vi "Fdx Create UDP Port (RX-CommPort).vi"(8 "error in":errorcluster, 9 "VlId":u16, 10 "CommPort Config":T2={"PortType"=enum."FDX_UDP_SAMPLING", "SubVIId"=1, "domainID"=1, "sideID"=1, "locationID"=1, "partitionID"=1, "UdpSrcPort"=1, "UdpDstPort"=1, "UdpNumBufMessages"=0, "UdpMaxMessageSize"=1000, "UdpSamplingRate"=0} {"partitionID" format="%.0b"}, 11 "port handle in":u32) -> (0 "error out":errorcluster, 1 "computedAddresses":T1 {"MACsrc" format="%.0x"}, 2 "commPort handle out":u32, 3 "port handle out":u32)   [LabVIEW 2020, in "AIM664LV.lvlib"]
doc: "This function creates a port to receive data from a specified UDP connection oriented port.\n\nThis function can be used only if the receiver is not running. This function assumes that FdxCmdRxVLControl was previously called in order to enable a VL for reception. On this VL this function creates an FDX communication Rx-port.\n\n<B>subVLid</B>: Not relevant in Rx Mode\n<B>UdpNumBuffMessages</B>: Number of messages which should be stored. For sampling port number should be set to 1, while for queuing port it should be set to adequate value. If set to 0, onboard target software will be set to a default value.\n<B>UdpMaxMessageSiize</B>: maximum size of the messsage to be received. For a sampling port, this is the fixed size of the sampling message, which means the size without the header overhead (MAC, IP and UDP).\nFor a queuing port this is the maximum size of the variable length message.\n(Queuing: 0..ize ? 8kBytes, Sampling: ul_UdpMaxMessageSize )\n<B>UdpSamplliingRate</B>: not relevant in RX mode"
uses:
  AIM664LV.lvlib
  _controls/comm_udp_rx.ctl
  _controls/comm_computedMAC-IP.ctl
  helpers/EthFrameManagement/controls/ip_src_info_afdx.ctl
  helpers/EthFrameManagement/EthFrameManagement.lvlib
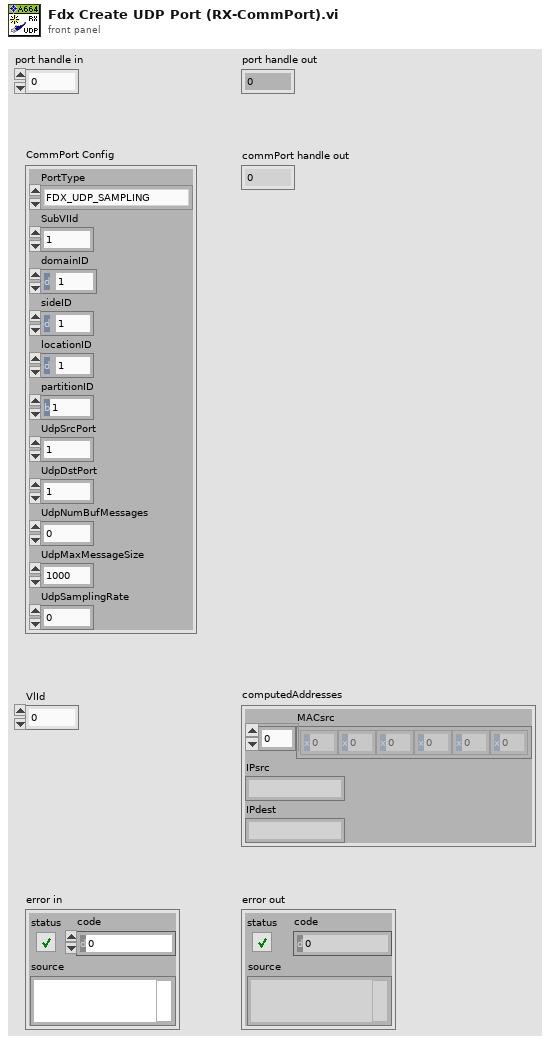
[diagram p1: front panel]
types:
  T1 = typedef "AIM664LV.lvlib/comm_computedMAC-IP.ctl" = cluster{"MACsrc":u8[], "IPsrc":string, "IPdest":string}
  T2 = typedef "AIM664LV.lvlib/comm_udp_rx.ctl" = cluster{"PortType":enum16{"FDX_UDP_SAMPLING", "FDX_UDP_QUEUING"}, "SubVIId":u32, "domainID":u8, "sideID":u8, "locationID":u8, "partitionID":u8, "UdpSrcPort":u16, "UdpDstPort":u16, "UdpNumBufMessages":u32, "UdpMaxMessageSize":u32, "UdpSamplingRate":u32}
  T3 = typedef "EthFrameManagement.lvlib/ip_src_info_afdx.ctl" = cluster{"domainID":u8, "sideID":u8, "locationID":u8, "partitionID":u8}
  T4 = cluster{"PortType":u32, "UdpSrc":u32, "IpSrc":u32, "VlId":u32, "IpDst":u32, "UdpDst":u32, "SubVlId":u32, "UdpNumBufMessages":u32, "UdpMaxMessageSize":u32, "UdpSamplingRate":u32}
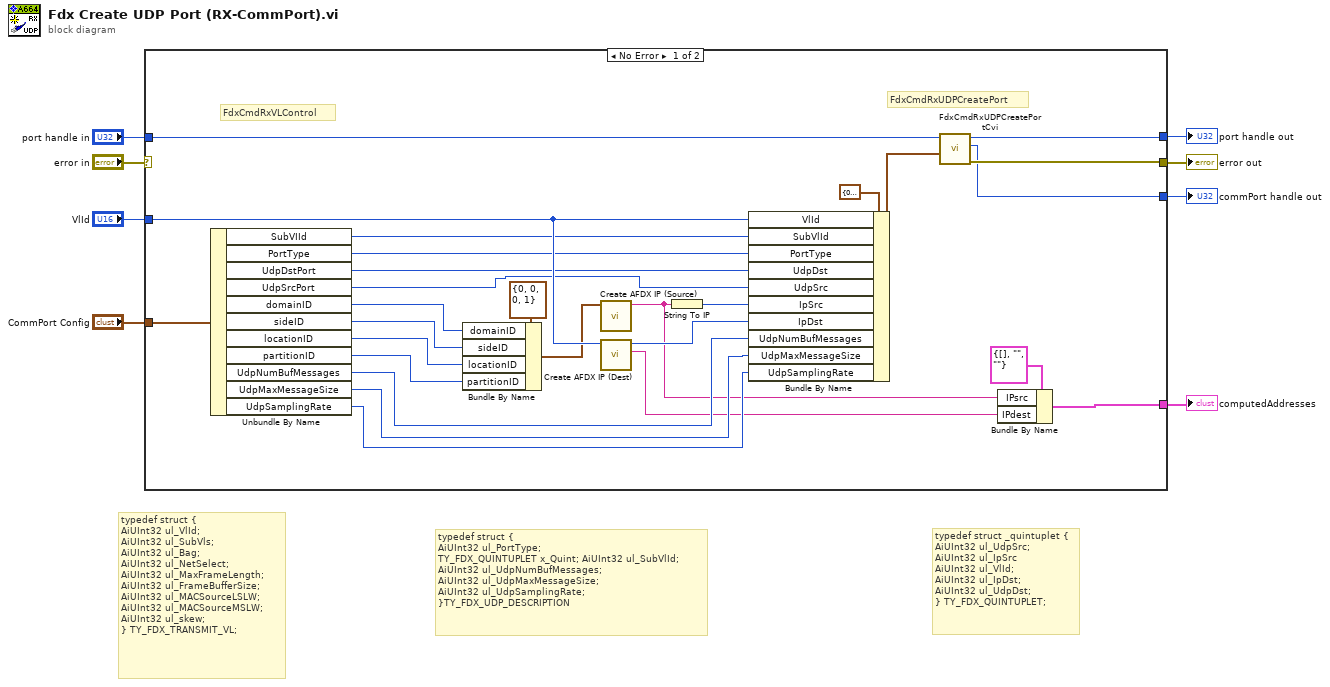
[diagram p0: block diagram]
diagram:
  # "typedef struct _quintuplet {\nAiUInt32 ul_UdpSrc;\nAiUInt32 ul_IpSrc\nAiUInt32 ul_VlId;\nAiUInt32 ul_IpDst;\nAiUInt32 ul_UdpDst;\n} TY_FDX_QUINTUPLET;"
  # "typedef struct {\nAiUInt32 ul_PortType;\nTY_FDX_QUINTUPLET x_Quint; AiUInt32 ul_SubVlId;\nAiUInt32 ul_UdpNumBufMessages;\nAiUInt32 ul_UdpMaxMessageSize;\nAiUInt32 ul_UdpSamplingRate;\n}TY_FDX_UDP_DESCRIPTION"
  # "typedef struct {\nAiUInt32 ul_VlId;\nAiUInt32 ul_SubVls;\nAiUInt32 ul_Bag;\nAiUInt32 ul_NetSelect;\nAiUInt32 ul_MaxFrameLength;\nAiUInt32 ul_FrameBufferSize;\nAiUInt32 ul_MACSourceLSLW;\nAiUInt32 ul_MACSourceMSLW;\nAiUInt32 ul_skew;\n} TY_FDX_TRANSMIT_VL;"
  n1 = case shown="No Error" "error in" {
    selector: "error in" -> [_ w36]
    tunnel: "port handle in" -> [w11 w37]
    tunnel: [w10 w37] -> w6
    tunnel: [w34 w36] -> w5
    tunnel: "CommPort Config" -> [w33 _]
    tunnel: [w35 _] -> w3
    tunnel: [w9 _] -> w2
    tunnel: "VlId" -> [w32 _]
    frame No Error {
      # "FdxCmdRxUDPCreatePort"
      # "FdxCmdRxVLControl"
      n2 = Unbundle By Name(w33) -> ("SubVIId"=w20:u32, "PortType"=w19:enum16{"FDX_UDP_SAMPLING", "FDX_UDP_QUEUING"}, "UdpDstPort"=w18:u16, "UdpSrcPort"=w17:u16, "domainID"=w24:u8, "sideID"=w23:u8, "locationID"=w22:u8, "partitionID"=w21:u8, "UdpNumBufMessages"=w16:u32, "UdpMaxMessageSize"=w15:u32, "UdpSamplingRate"=w14:u32)
      n3 = Bundle By Name(cluster=T3 {"domainID"=0, "sideID"=0, "locationID"=0, "partitionID"=1} ("Source Info"), "domainID"=w24, "sideID"=w23, "locationID"=w22, "partitionID"=w21) -> (w25:T3)
      n4 = call "Create AFDX IP (Source).vi"("Source Info"=w25) -> ("ip address"=w13:string)  [unwired: 10 in]
      n5 = call "Create AFDX IP (Dest).vi"("VL"=w32) -> ("ip string"=w12:string, "ip net"=w27:u32)  [unwired: 9 in]
      n6 = String To IP(1:w13) -> (0:w28:u32)
      n7 = Bundle By Name(cluster=T4 {"PortType"=0, "UdpSrc"=0, "IpSrc"=0, "VlId"=0, "IpDst"=0, "UdpDst"=0, "SubVlId"=0, "UdpNumBufMessages"=0, "UdpMaxMessageSize"=0, "UdpSamplingRate"=0} ("UdpDescription"), "VlId"=w32, "SubVlId"=w20, "PortType"=w19, "UdpDst"=w18, "UdpSrc"=w17, "IpSrc"=w28, "IpDst"=w27, "UdpNumBufMessages"=w16, "UdpMaxMessageSize"=w15, "UdpSamplingRate"=w14) -> (w29:T4)
      n8 = call "FdxCmdRxUDPCreatePortCvi.vi"("UdpDescription"=w29, "InstrumentHandle_port"=w11) -> ("error out"=w34:errorcluster, "UdpHandle"=w9:u32, "InstrumentHandle_port"=w10:u32)  [unwired: 7 in]
      n9 = Bundle By Name(cluster=T1 {"MACsrc"=[], "IPsrc"="", "IPdest"=""} ("computedAddresses"), "IPsrc"=w13, "IPdest"=w12) -> (w35:T1)
    }
    frame Error {
    }
  }
  "port handle out" <- w6
  "commPort handle out" <- w2
  "error out" <- w5
  "computedAddresses" <- w3
